vi "Configuration-Product.vi"(3 "error in":errorcluster) -> (0 "error out":errorcluster)   [LabVIEW 2015]
uses:
  Control Button/Exit.ctl
panel:
  in  "Load Old Configuration":bool caption="Save Configuration"
  in  "Save New Configuration":bool caption="Save Configuration"
  in  "Quit":T1
  in  "Product Configuration":string[][](table)
  out "Array":string[](array[string])
  # "Product Configuration"
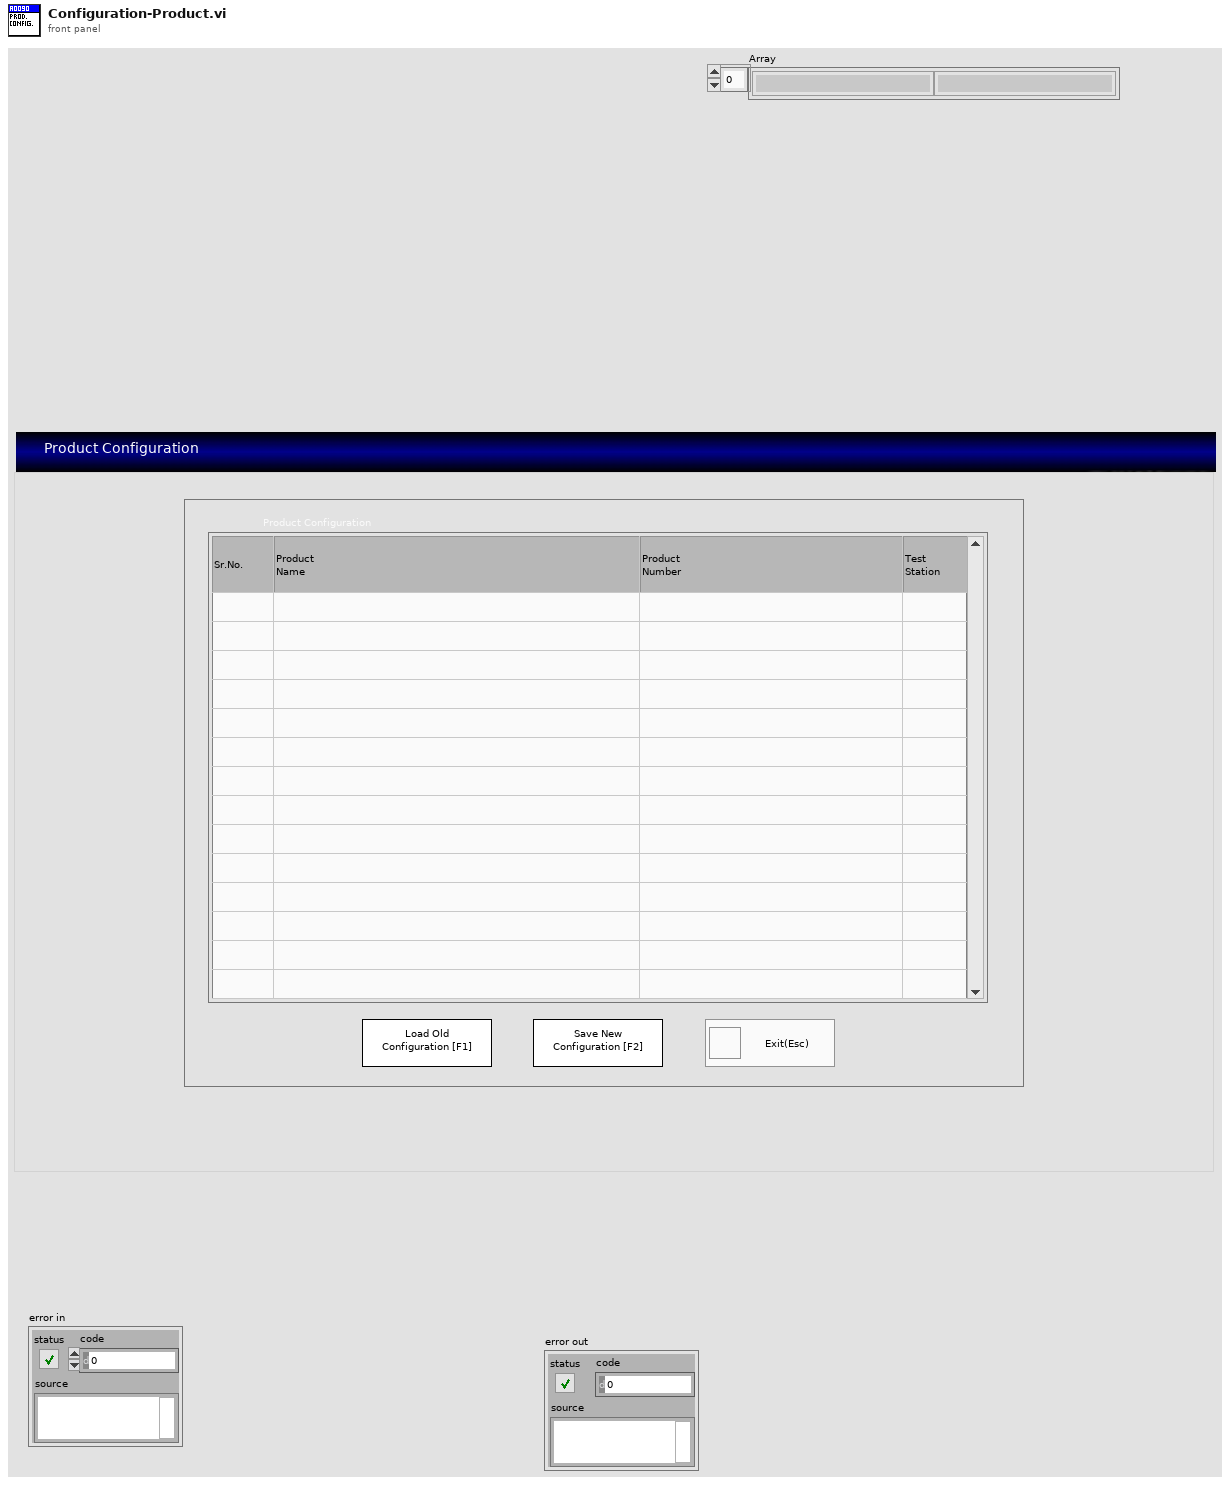
[diagram p1: front panel]
types:
  T1 = typedef "Exit.ctl" = bool
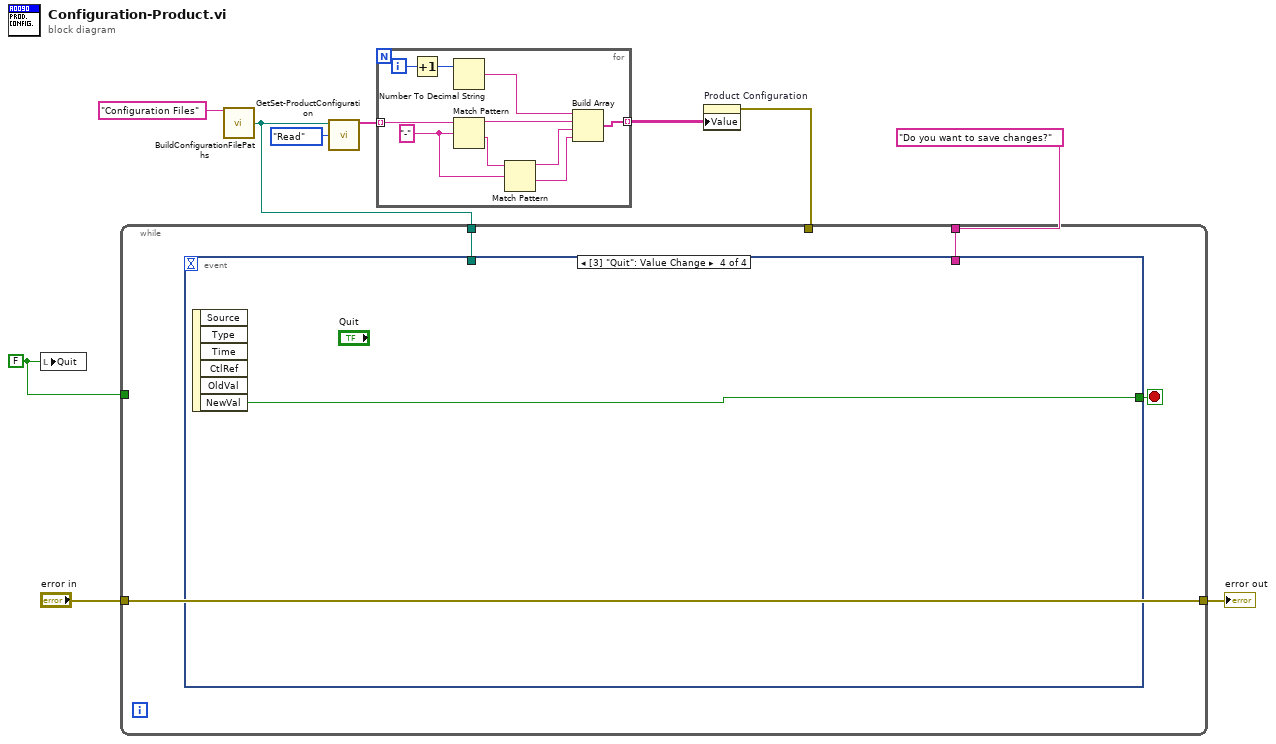
[diagram p0: block diagram]
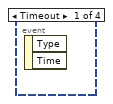
[diagram p2: hidden frame]
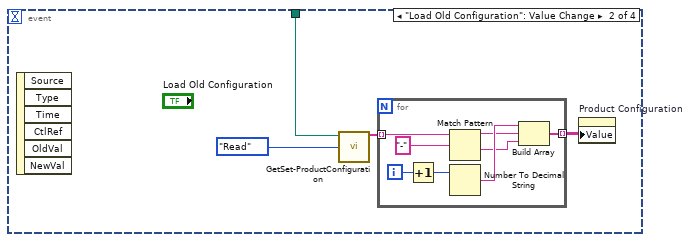
[diagram p3: hidden frame]
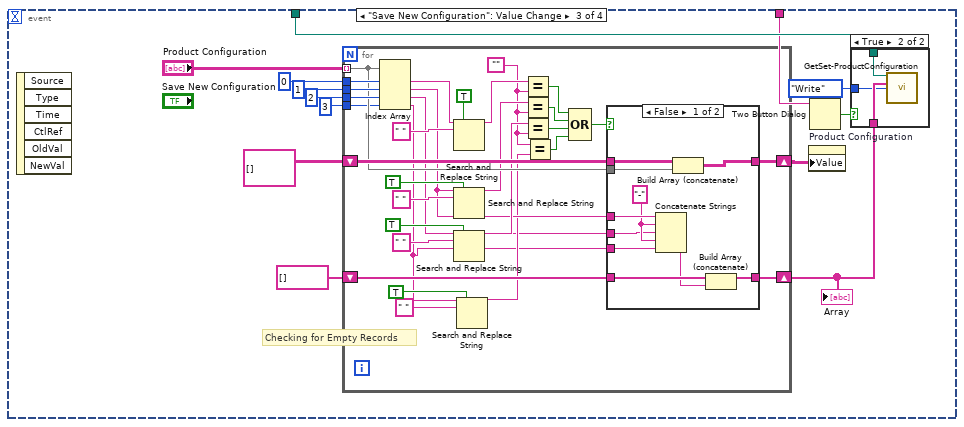
[diagram p4: hidden frame]
diagram:
  w1 = T1 FALSE ("Quit")
  n1 = local write "Quit"(w1) -> ()
  n2 = call "BuildConfigurationFilePaths.vi"("name or relative path"="Configuration Files") -> ("Product Configuration"=w7:path)  [unwired: 10 in, 4 out]
  n3 = call "GetSet-ProductConfiguration.vi"("Filepath"=w7, "Read/Write"=enum16{"Read", "Write"}."Read") -> ("Product Configuration Out"=w9:string[])  [unwired: 12 in, 1 out]
  n4 = for {
    tunnel: w9 -> [w16] mode=indexing
    tunnel: [w20] -> w5 mode=indexing
    i -> [w19]
    w14 = "-" ("regular expression")
    n5 = Increment(x=w19) -> (x+1=w18:i32)
    n6 = Number To Decimal String(number=w18) -> (decimal integer string=w17:string)  [unwired: 1 in]
    n7 = Match Pattern(string=w16, regular expression=w14) -> (before substring=w15:string, after substring=w13:string)  [unwired: 1 in, 2 out]
    n8 = Match Pattern(string=w13, regular expression=w14) -> (before substring=w12:string, after substring=w11:string)  [unwired: 1 in, 2 out]
    n9 = Build Array(w17, w15, w12, w11) -> (w20:string[])
  }
  n10 = property on="Product Configuration" class="Tbl (strict)"("Value"=w5) -> (error out=w6:errorcluster)  [unwired: 2 in, 1 out]
  n11 = while {
    tunnel: w7 -> [w23]
    tunnel: "Do you want to save changes?" ("message") -> [w22]
    tunnel: w6 -> [_]
    tunnel: "error in" -> [w21]
    tunnel: [w21] -> w2
    tunnel: w1 -> [_]
    stop <- w24 stop-if-true
    n12 = event shown="[3] \"Quit\": Value Change" {
      selector: _ -> [_ _ _ _]
      dyn-events: _ -> [_ _ _ _]
      timeout: _ -> [_ _ _ _]
      tunnel: [_ _ _ w96] -> w24
      tunnel: w23 -> [_ w28 w49 _]
      tunnel: w22 -> [_ _ w39 _]
      event Timeout {
        n13 = event-data() -> ()  [unwired: 1 in, 2 out]
      }
      event "Load Old Configuration": Value Change {
        n14 = event-data() -> ()  [unwired: 1 in, 6 out]
        n15 = call "GetSet-ProductConfiguration.vi"("Filepath"=w28, "Read/Write"=enum16{"Read", "Write"}."Read") -> ("Product Configuration Out"=w26:string[])  [unwired: 12 in, 1 out]
        n16 = for {
          tunnel: w26 -> [w32] mode=indexing
          tunnel: [w36] -> w25 mode=indexing
          i -> [w35]
          n17 = Increment(x=w35) -> (x+1=w34:i32)
          n18 = Match Pattern(string=w32, regular expression="-") -> (before substring=w29:string, after substring=w30:string)  [unwired: 1 in, 2 out]
          n19 = Number To Decimal String(number=w34) -> (decimal integer string=w33:string)  [unwired: 1 in]
          n20 = Build Array(w33, w29, w30) -> (w36:string[])
        }
        n21 = property on="Product Configuration" class="Tbl (strict)"("Value"=w25) -> ()  [unwired: 2 in, 2 out]
      }
      event "Save New Configuration": Value Change {
        # "Checking for Empty Records"
        n22 = event-data() -> ()  [unwired: 1 in, 6 out]
        n23 = for {
          tunnel: "Product Configuration" -> [w73] mode=indexing
          tunnel: 0 ("index") -> [w80]
          tunnel: 1 ("index") -> [w79]
          tunnel: 2 ("index") -> [w78]
          shift-right: [w72] -> w38
          shift-left: string[][] [] -> [w74]
          shift-right: [w59] -> w41
          shift-left: string[] [] -> [w60]
          tunnel: 3 ("index") -> [w57]
          w54 = ""
          n24 = Index Array(array=w73, index #1=w80, index #2=w79, index #3=w78, index #4=w57) -> (element #1=w68:string, element #2=w58:string, element #3=w51:string, element #4=w50:string)
          n25 = Search and Replace String(replace all?=TRUE ("replace all? (F)"), input string=w68, search string=" ") -> (result string=w67:string)  [unwired: 5 in, 3 out]
          n26 = Search and Replace String(replace all?=TRUE ("replace all? (F)"), input string=w58, search string=" ") -> (result string=w61:string)  [unwired: 5 in, 3 out]
          n27 = Search and Replace String(replace all?=TRUE ("replace all? (F)"), input string=w51, search string=" ") -> (result string=w62:string)  [unwired: 5 in, 3 out]
          n28 = Search and Replace String(replace all?=TRUE ("replace all? (F)"), input string=w50, search string=" ") -> (result string=w53:string)  [unwired: 5 in, 3 out]
          n29 = Equal?(x=w67, y=w54) -> (x = y?=w77:bool)
          n30 = Equal?(x=w61, y=w54) -> (x = y?=w76:bool)
          n31 = Equal?(x=w62, y=w54) -> (x = y?=w75:bool)
          n32 = Equal?(x=w54, y=w53) -> (x = y?=w52:bool)
          n33 = Compound Arithmetic op=OR(w77, w76, w75, w52) -> (w71:bool)
          n34 = case shown="False" w71 {
            tunnel: w74 -> [w90 w92]
            tunnel: w73 -> [w89 _]
            tunnel: [w88 w92] -> w72
            tunnel: w60 -> [w87 w91]
            tunnel: [w86 w91] -> w59
            tunnel: w58 -> [w85 _]
            tunnel: w51 -> [w82 _]
            tunnel: w50 -> [w81 _]
            frame False {
              w83 = "-" ("string")
              n35 = Concatenate Strings(w85, w83, w82, w83, w81) -> (w84:string)
              n36 = Build Array (concatenate)(w90, w89) -> (w88:string[][])
              n37 = Build Array (concatenate)(w87, w84) -> (w86:string[])
            }
            frame True {
            }
          }
        }
        "Array" <- w41
        n38 = property on="Product Configuration" class="Tbl (strict)"("Value"=w38) -> ()  [unwired: 2 in, 2 out]
        n39 = Two Button Dialog(message=w39) -> (T button?=w48:bool)  [unwired: 2 in]
        n40 = case shown="True" w48 {
          tunnel: w49 -> [_ w95]
          tunnel: w41 -> [_ w94]
          tunnel: enum16{"Read", "Write"}."Write" ("Read/Write") -> [_ w93]
          frame False {
          }
          frame True {
            n41 = call "GetSet-ProductConfiguration.vi"("Filepath"=w95, "Product Configuration In"=w94, "Read/Write"=w93) -> ()  [unwired: 11 in, 2 out]
          }
        }
      }
      event Value Change {
        n42 = event-data() -> ("NewVal"=w96:T1)  [unwired: 1 in, 5 out]
      }
    }
  }
  "error out" <- w2
